vi "myRIO_BRig_RT__Case_Exp_subState_LC__Cue1.vi"(7 "input_spout":enum16{"Left", "Right"}(ring), 8 "input_dataCurrent":u16[](array[numeric]), 10 "input_dataLC":u16[](array[numeric])) -> (1 "output_LC_led":bool, 2 "output_LC":bool)   [LabVIEW 2014]
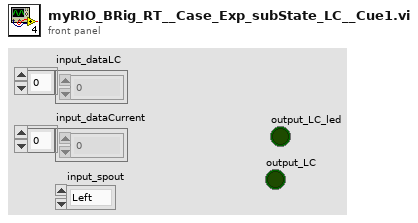
[diagram p1: front panel]
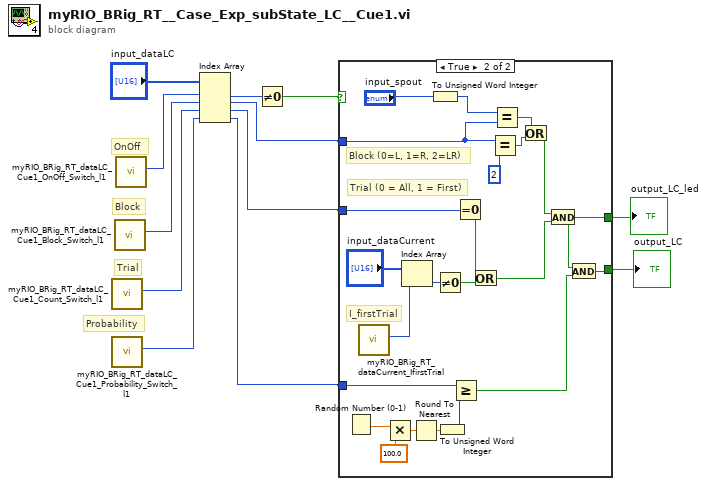
[diagram p0: block diagram]
diagram:
  # "Probability"
  # "Trial"
  # "Block"
  # "OnOff"
  n1 = call "myRIO_BRig_RT_dataLC_Cue1_Count_Switch_l1.vi"() -> ("output_Cue1_l1_First_Count"=w9:i32)  [unwired: 11 in]
  n2 = call "myRIO_BRig_RT_dataLC_Cue1_Probability_Switch_l1.vi"() -> ("output_Cue1_l1_First_Probability"=w8:i32)  [unwired: 11 in]
  n3 = call "myRIO_BRig_RT_dataLC_Cue1_Block_Switch_l1.vi"() -> ("output_Cue1_l1_First_Block"=w10:i32)  [unwired: 11 in]
  n4 = call "myRIO_BRig_RT_dataLC_Cue1_OnOff_Switch_l1.vi"() -> ("output_Cue1_l1_First_OnOff"=w11:i32)  [unwired: 11 in]
  n5 = Index Array(array="input_dataLC", index #1=w11, index #2=w10, index #3=w9, index #4=w8) -> (element #1=w7:u16, element #2=w5:u16, element #3=w4:u16, element #4=w3:u16)
  n6 = Not Equal To 0?(x=w7) -> (x != 0?=w6:bool)
  n7 = case shown="True" w6 {
    tunnel: w5 -> [_ w19]
    tunnel: w4 -> [_ w20]
    tunnel: w3 -> [_ w21]
    tunnel: [_ w15] -> w2
    tunnel: [_ w13] -> w1
    frame False {
    }
    frame True {
      # "Block (0=L, 1=R, 2=LR)"
      # "Trial (0 = All, 1 = First)"
      # "I_firstTrial"
      n8 = Random Number (0-1)() -> (number: 0 to 1=w28:dbl)
      n9 = call "myRIO_BRig_RT_dataCurrent_IfirstTrial.vi"() -> ("output_I_firstTrial"=w32:i32)  [unwired: 11 in]
      n10 = Multiply(x=w28, y=100.0) -> (x*y=w27:dbl)
      n11 = Index Array(array="input_dataCurrent", index=w32) -> (element=w31:u16)
      n12 = Round To Nearest(number=w27) -> (nearest integer value=w26:dbl)
      n13 = To Unsigned Word Integer(number="input_spout") -> (unsigned 16bit integer=w18:u16)
      n14 = Not Equal To 0?(x=w31) -> (x != 0?=w29:bool)
      n15 = To Unsigned Word Integer(number=w26) -> (unsigned 16bit integer=w25:u16)
      n16 = Greater Or Equal?(x=w21, y=w25) -> (x >= y?=w14:bool)
      n17 = Equal To 0?(x=w20) -> (x = 0?=w30:bool)
      n18 = Or(x=w30, y=w29) -> (x .or. y?=w16:bool)
      n19 = Equal?(x=w19, y=u16 2) -> (x = y?=w33:bool)
      n20 = Equal?(x=w18, y=w19) -> (x = y?=w34:bool)
      n21 = Or(x=w34, y=w33) -> (x .or. y?=w17:bool)
      n22 = And(x=w17, y=w16) -> (x .and. y?=w13:bool)
      n23 = And(x=w13, y=w14) -> (x .and. y?=w15:bool)
    }
  }
  "output_LC" <- w2
  "output_LC_led" <- w1
